vi "CameraSetParams.vi"(8 "error in (no error)":errorcluster, 10 "settings":T2={"exposure"=0.0, "external"=FALSE, "roi"={"left"=0, "top"=0, "right"=0, "bottom"=0}, "frames"=0, "binning"={"x"=1, "y"=1}}, 11 "NIvision in":refnum<class "IMAQdx_Flea3_Firewire.lvclass">) -> (0 "error out":errorcluster, 1 "roi_out":T1, 2 "attributes":variant[](array[variant]), 3 "NIvision out":refnum<class "IMAQdx_Flea3_Firewire.lvclass">)   [LabVIEW 2012, in "IMAQdx_Flea3_Firewire.lvclass"]
uses:
  <userlib>/BIAS2/classes/IMAQdx_Flea3_Firewire/IMAQdx_Flea3_Firewire.lvclass
  <userlib>/BIAS2/subvis/ExposureSettings.ctl
  <userlib>/BIAS2/subvis/ROI_rect.ctl
  <vilib>/vision/driver/IMAQdx.llb/IMAQdx Acquisition Mode.ctl
  <userlib>/BIAS2/classes/IMAQdx_Flea3_Firewire/IMAQdx_Flea3_Firewire.lvclass/IMAQdx_Flea3_Firewire.ctl
  <vilib>/vision/driver/NI_Vision_Acquisition_Software.lvlib
  <resource>/objmgr/imaqdx.rc
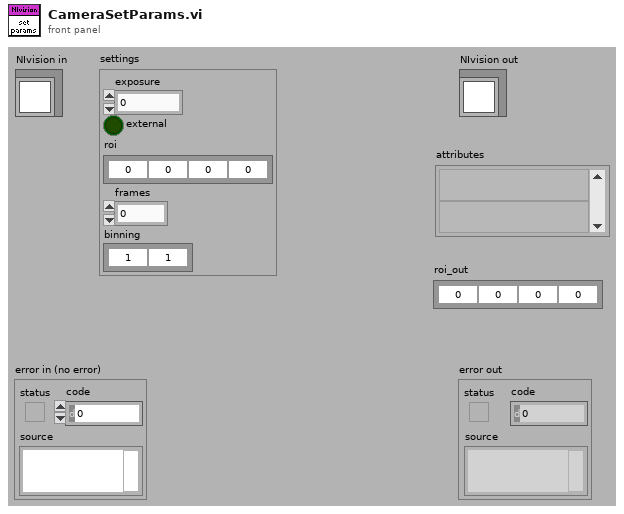
[diagram p1: front panel]
types:
  T1 = typedef "ROI_rect.ctl" = cluster{"left":i32, "top":i32, "right":i32, "bottom":i32}
  T2 = typedef "ExposureSettings.ctl" = cluster{"exposure":dbl, "external":bool, "roi":T1, "frames":i32, "binning":cluster{"x":u8, "y":u8}}
  T3 = typedef "NI_Vision_Acquisition_Software.lvlib/IMAQdx Acquisition Mode.ctl" = enum32{"One Shot", "Continuous"}
  T4 = typedef "IMAQdx.ctl" = refnum<k21>
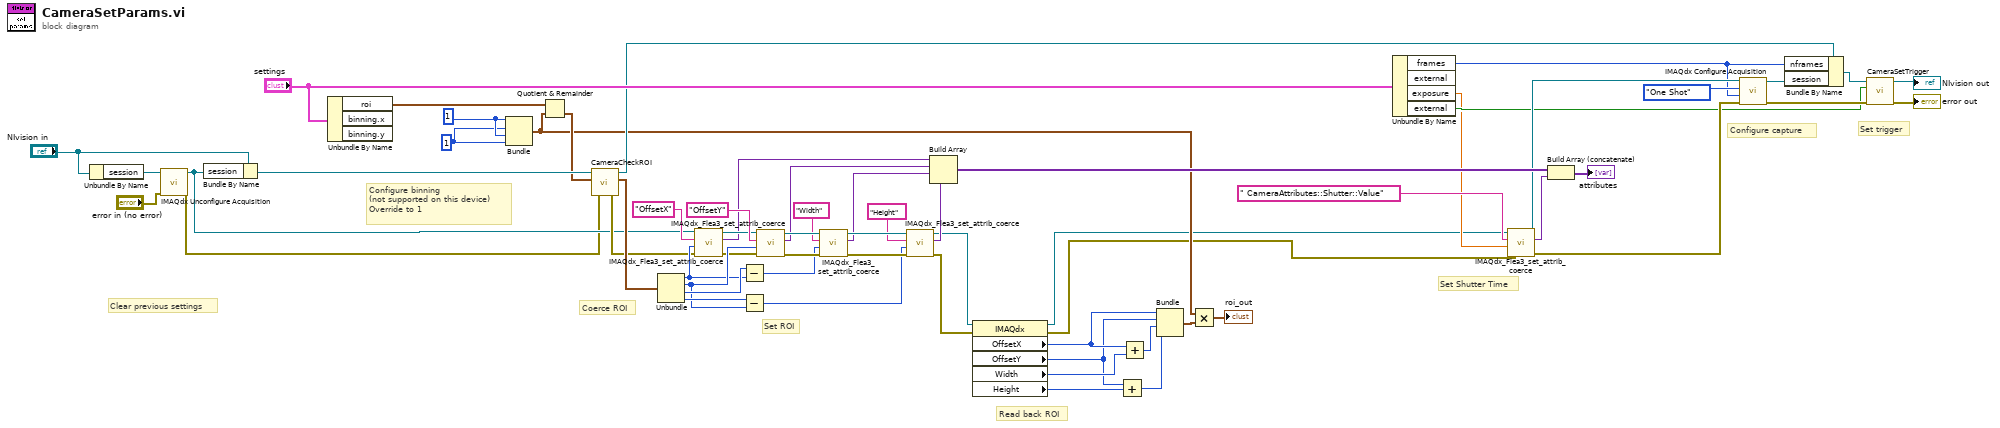
[diagram p0: block diagram]
diagram:
  w4 = 1
  w5 = 1
  # "Set trigger"
  # "Configure capture"
  # "Set Shutter Time"
  # "Read back ROI"
  # "Set ROI"
  # "Coerce ROI"
  # "Clear previous settings"
  # "Configure binning\n(not supported on this device)\nOverride to 1"
  n1 = Unbundle By Name("NIvision in") -> ("session"=w29:refnum<k21>)
  n2 = call <vilib>:"IMAQdx Unconfigure Acquisition.vi"("error in"="error in (no error)", "Session In"=w29) -> ("error out"=w6:errorcluster, "Session Out"=w7:T4)  [unwired: 8 in]
  n3 = Bundle By Name(cluster="NIvision in", "session"=w7) -> (w14:refnum<class "IMAQdx_Flea3_Firewire.lvclass">)
  n4 = Unbundle By Name("settings") -> ("roi"=w12:T1)  [unwired: 2 out]
  n5 = Bundle(w5, w4, w5, w4) -> (w8:cluster{i32, i32, i32, i32})  [unwired: 1 in]
  n6 = Quotient & Remainder(x=w12, y=w8) -> (floor(x/y)=w11:T1)  [unwired: 1 out]
  n7 = call-dynamic "CameraCheckROI.vi"("error in (no error)"=w6, "ROI_in"=w11, "IMAQdx in"=w14) -> ("error out"=w16:errorcluster, "ROI_out"=w17:T1, "IMAQdx out"=w18:refnum<class "IMAQdx_Flea3_Firewire.lvclass">)  [unwired: 6 in]
  n8 = Unbundle(w17) -> ("left"=w53:i32, "top"=w57:i32, "right"=w62:i32, "bottom"=w60:i32)
  n9 = call <userlib>:"IMAQdx_Flea3_set_attrib_coerce.vi"("error in"=w16, "value"=w53, "attribute"="OffsetX", "IMAQdx in"=w7) -> ("error out"=w56:errorcluster, "attrib out"=w54:variant, "IMAQdx out"=w55:T4)  [unwired: 1 out]
  n10 = Subtract(x=w62, y=w53) -> (x-y=w48:i32)
  n11 = Subtract(x=w60, y=w57) -> (x-y=w47:i32)
  n12 = call <userlib>:"IMAQdx_Flea3_set_attrib_coerce.vi"("error in"=w56, "value"=w57, "attribute"="OffsetY", "IMAQdx in"=w55) -> ("error out"=w51:errorcluster, "attrib out"=w46:variant, "IMAQdx out"=w52:T4)  [unwired: 1 out]
  n13 = call <userlib>:"IMAQdx_Flea3_set_attrib_coerce.vi"("error in"=w51, "value"=w48, "attribute"="Width", "IMAQdx in"=w52) -> ("error out"=w49:errorcluster, "attrib out"=w45:variant, "IMAQdx out"=w50:T4)  [unwired: 1 out]
  n14 = call <userlib>:"IMAQdx_Flea3_set_attrib_coerce.vi"("error in"=w49, "value"=w47, "attribute"="Height", "IMAQdx in"=w50) -> ("error out"=w33:errorcluster, "attrib out"=w44:variant, "IMAQdx out"=w32:T4)  [unwired: 1 out]
  n15 = Build Array(w54, w46, w45, w44) -> (w41:variant[])
  n16 = property class="IMAQdx"(reference=w32, error in=w33) -> (reference out=w1:T4, error out=w2:errorcluster, "OffsetX"=w38:u32, "OffsetY"=w37:u32, "Width"=w39:u32, "Height"=w40:u32)
  n17 = Add(x=w37, y=w40) -> (x+y=w35:u32)
  n18 = Add(x=w38, y=w39) -> (x+y=w36:u32)
  n19 = Bundle("OffsetX"=w38, "OffsetY"=w37, w36, w35) -> (w10:cluster{"OffsetX":u32, "OffsetY":u32, u32, u32})  [unwired: 1 in]
  n20 = Multiply(x=w8, y=w10) -> (x*y=→"roi_out":cluster{u32, u32, u32, u32})
  n21 = Unbundle By Name("settings") -> ("frames"=w20:i32, "exposure"=w3:dbl, "external"=w13:bool)  [unwired: 1 out]
  n22 = call <userlib>:"IMAQdx_Flea3_set_attrib_coerce.vi"("error in"=w2, "value"=w3, "attribute"=" CameraAttributes::Shutter::Value" ("ActiveAttribute"), "IMAQdx in"=w1) -> ("error out"=w22:errorcluster, "attrib out"=w30:variant, "IMAQdx out"=w24:T4)  [unwired: 1 out]
  n23 = Build Array (concatenate)(w41, w30) -> (→"attributes":variant[])
  n24 = call <vilib>:"IMAQdx Configure Acquisition.vi"("error in"=w22, "Number of Buffers"=w20, "Continuous?"=IMAQdx_Acquisition_Mode."One Shot", "Session In"=w24) -> ("error out"=w21:errorcluster, "Session Out"=w25:T4)  [unwired: 6 in]
  n25 = Bundle By Name(cluster=w18, "nframes"=w20, "session"=w25) -> (w15:refnum<class "IMAQdx_Flea3_Firewire.lvclass">)
  n26 = call-dynamic "CameraSetTrigger.vi"("error in (no error)"=w21, "external?"=w13, "IMAQdx in"=w15) -> ("error out"=→"error out":errorcluster, "IMAQdx out"=→"NIvision out":refnum<class "IMAQdx_Flea3_Firewire.lvclass">)  [unwired: 6 in, 1 out]
